vi "JKISM++ Array Parameter Status.vi"() -> (1 "Active Read Oper":T1, 2 "Active Write Oper":T1, 4 "cache size":i32)   [LabVIEW 2020, in "JKISM++ MassData Parameter Support.lvlib"]
doc: "Convert complex argument(variant) to hex string, which could be safely used as state argument without broking the string queue logic.\n\n<b>Inputs:</b>\n - <b>Variant</b>: Complex data in variant format.\n\n<b>Outputs:</b>\n - <b>HEX String (0-9,A-F)</b>: Hex String, which contains no invisible string following JKISM's rule"
uses:
  JKISM++ MassData Parameter Support.lvlib
  _support/Def-MassDataOper-Status.ctl
  _support/Operation-FGV-MassData.ctl
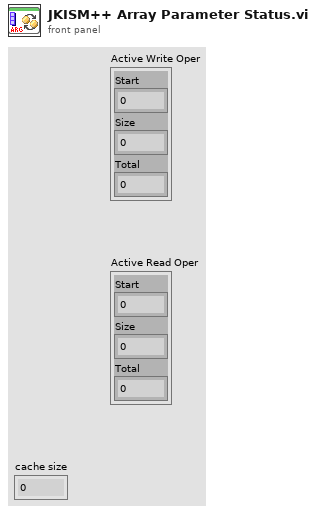
[diagram p1: front panel]
types:
  T1 = typedef "JKISM++ MassData Parameter Support.lvlib/Def-MassDataOper-Status.ctl" = cluster{"Start":i32, "Size":i32, "Total":i32}
  T2 = typedef "JKISM++ MassData Parameter Support.lvlib/Operation-FGV-MassData.ctl" = enum16{"Initialize", "Read", "Write", "Status", "Release"}
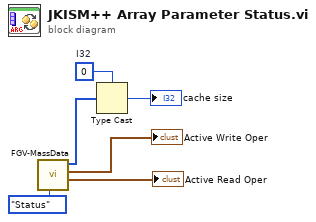
[diagram p0: block diagram]
diagram:
  w1 = 0  # I32
  n1 = call "FGV-MassData.vi"("Operation"=Operation-FGV-MassData."Status") -> ("Active Read Oper"=→"Active Read Oper":T1, "Active Write Oper"=→"Active Write Oper":T1, "Data out"=w3:u8[])  [unwired: 7 in, 1 out]
  n2 = Type Cast(type=w1, x=w3) -> (*(type *) &x=→"cache size":i32)
